vi "start.vi"(8 "error in (no error)":errorcluster, 9 "ILCAppConfig":T1={"ILCConfig"={"Input Channels"=enum."Channel 0", "Scan Rate (Hz) "=enum."50", "ADC PGA Gain"=0}, "RS232Config"={"VISA resource name"="", "Baud Rate"=9600, "Data Bits"=8, "Parity"=enum."None", "Stop Bits"=10, "Flow Control"=0, "Timeout (ms)"=10000}, "Application Timing"={"Loop Period (ms)"=1}} {"Application Timing"."Loop Period (ms)" min=1 max=5000; "RS232Config"."Stop Bits" items=["1.0"=10, "1.5"=15, "2.0"=20]; "RS232Config"."Flow Control" items=["None", "XON/XOFF", "RTS/CTS", "XON/XOFF & RTS/CTS", "DTR/DSR", "XON/XOFF & DTR/DSR"]; "RS232Config"."Data Bits" min=5 max=8 step=1; "ILCConfig"."ADC PGA Gain" max=7}, 10 "model":refnum<class "Model.lvclass">, 11 "StandbyState in":refnum<class "StandbyState.lvclass">) -> (0 "error out":errorcluster, 2 "model 2":refnum<class "Model.lvclass">, 3 "StandbyState out":refnum<class "StandbyState.lvclass">)   [LabVIEW 2012, in "StandbyState.lvclass"]
uses:
  StandbyState.lvclass
  Model/Model/Model.lvclass
  State/ILCAppConfig.ctl
  Configuration/ILCConfig.ctl
  Configuration/InputChannels.ctl
  Configuration/ScanRate_Hz_MultichannelOptions.ctl
  Configuration/RS232Config.ctl
  Model/Model/ApplicationTiming.ctl
  Typedefs/StateSelector.ctl
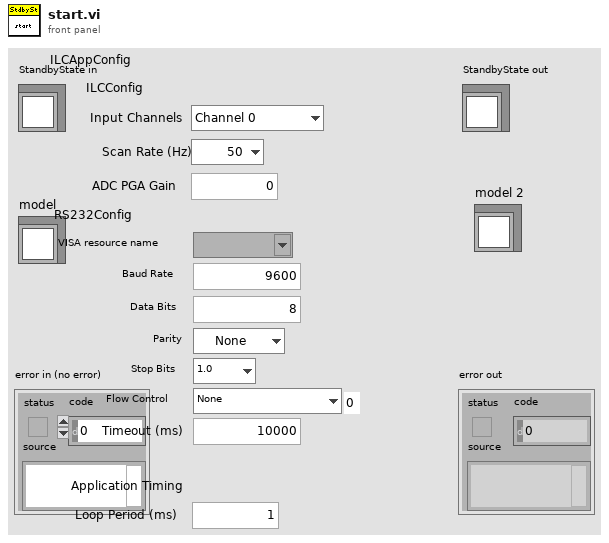
[diagram p1: front panel]
types:
  T1 = typedef "ILCAppConfig.ctl" = cluster{"ILCConfig":T2, "RS232Config":T5, "Application Timing":T6}
  T2 = typedef "ILCConfig.ctl" = cluster{"Input Channels":T3, "Scan Rate (Hz) ":T4, "ADC PGA Gain":u8}
  T3 = typedef "InputChannels.ctl" = enum16{"Channel 0", "3 Channels", "5 Channels"}
  T4 = typedef "ScanRate_Hz_MultichannelOptions.ctl" = enum16{"50", "60", "100", "120", "200", "240", "300", "400", "480", "600", "1200", "2400", "4800"}
  T5 = typedef "RS232Config.ctl" = cluster{"VISA resource name":refnum<visa-resource-name>, "Baud Rate":u32, "Data Bits":u16, "Parity":enum16{"None", "Odd", "Even", "Mark", "Space"}, "Stop Bits":u16, "Flow Control":u16, "Timeout (ms)":u32}
  T6 = typedef "ApplicationTiming.ctl" = cluster{"Loop Period (ms)":u16}
  T7 = typedef "StateSelector.ctl" = enum16{"DataOnDemandState", "DataStreamingState", "FaultState", "OffState", "StandbyState"}
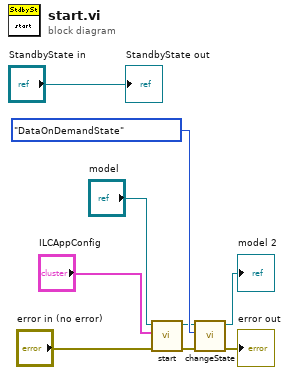
[diagram p0: block diagram]
diagram:
  n1 = call "start.vi"("error in (no error)"="error in (no error)", "ILCAppConfig"="ILCAppConfig", "Model in"="model") -> ("error out"=w2:errorcluster, "Model out"=w6:refnum<class "Model.lvclass">)  [unwired: 7 in]
  n2 = call "changeState.vi"("error in (no error)"=w2, "State:"=StateSelector."DataOnDemandState", "Model in"=w6) -> ("error out"=→"error out":errorcluster, "Model out"=→"model 2":refnum<class "Model.lvclass">)  [unwired: 7 in]
  "StandbyState out" <- "StandbyState in"
